vi "纳清探头一键校准.vi"(4 "校准量程":u16, 5 "校准方式":u16, 6 "MB_Master输入":refnum<class "MB_Master.lvclass">, 7 "探头":T1(ring), 8 "error in (no error)":errorcluster caption="错误输入（无错误）", 9 "标液三":cluster{"标准值":sgl, "检测值":sgl, "原始值":sgl}, 10 "标液二":cluster{"标准值":sgl, "检测值":sgl, "原始值":sgl}, 11 "标液一":cluster{"标准值":sgl, "检测值":sgl, "原始值":sgl}) -> (0 "error out":errorcluster caption="错误输出")   [LabVIEW 2016, in "斯坦道多参数.lvlib"]
uses:
  <vilib>/Plasmionique/MB Master/MB_Master/MB_Master.lvclass
  <vilib>/Plasmionique/MB Master/MB Master.lvlib
panel:
  out "数组":u16[](array[numeric]) format="%04x"
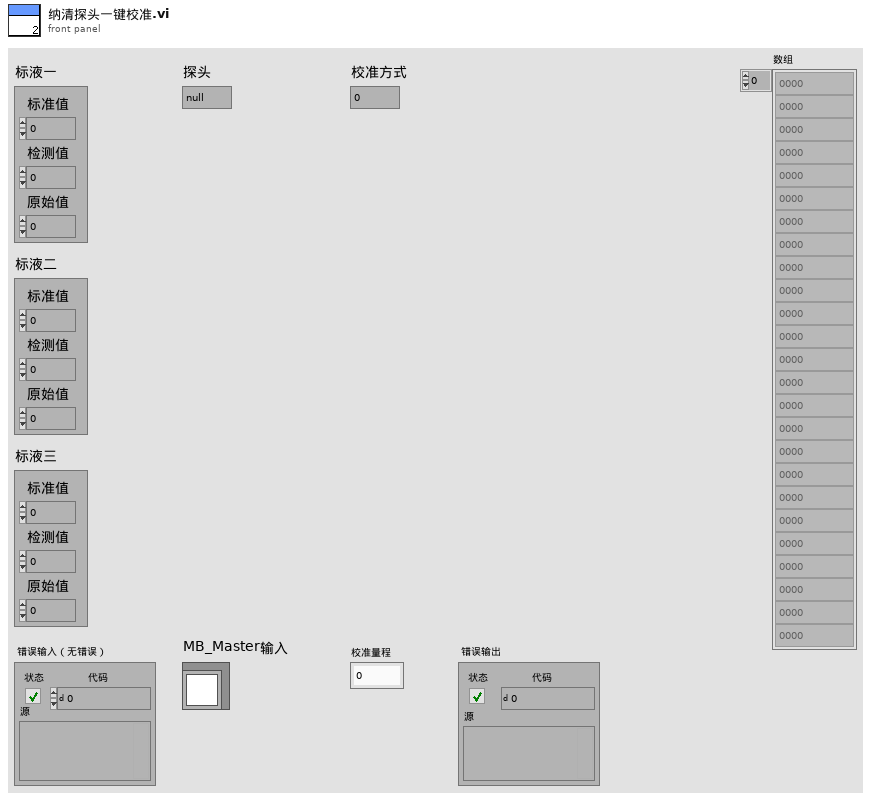
[diagram p1: front panel]
types:
  T1 = enum16{"null", "pH", "DO", "浊度", "电导率", "叶绿素a", "藻密度", "氨氮"}
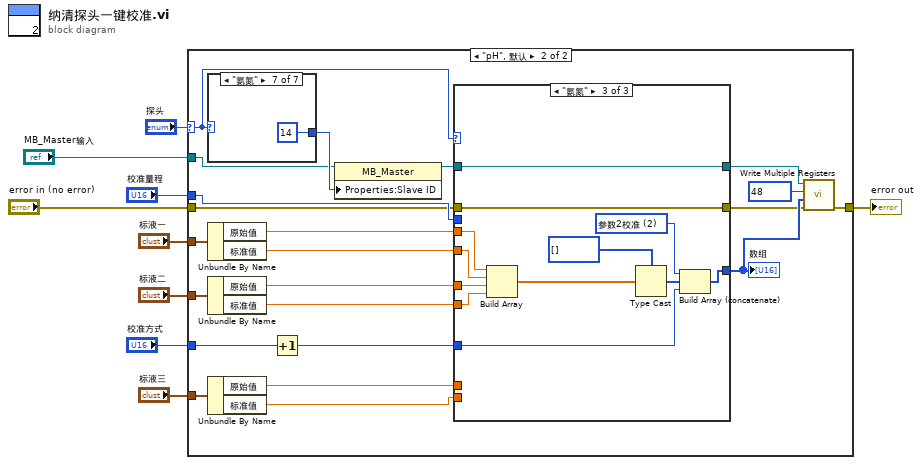
[diagram p0: block diagram]
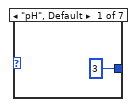
[diagram p3: hidden frame]
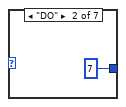
[diagram p4: hidden frame]
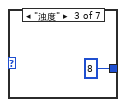
[diagram p5: hidden frame]
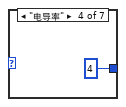
[diagram p6: hidden frame]
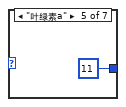
[diagram p7: hidden frame]
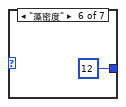
[diagram p8: hidden frame]
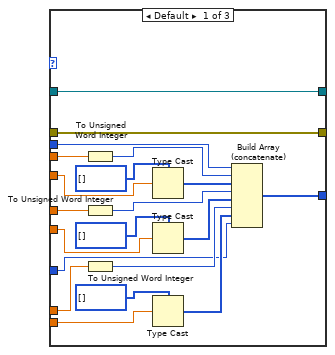
[diagram p9: hidden frame]
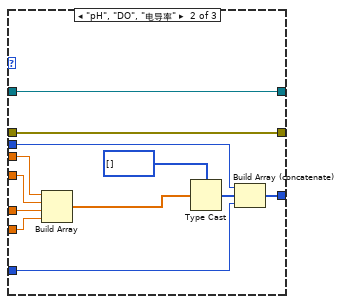
[diagram p10: hidden frame]
diagram:
  n1 = case shown="\"pH\", 默认" "探头" {
    selector: "探头" -> [_ w17]
    tunnel: "error in (no error)" -> [w10 w12]
    tunnel: [w10 w32] -> w8
    tunnel: "标液一" -> [_ w31]
    tunnel: "标液二" -> [_ w30]
    tunnel: "标液三" -> [_ w29]
    tunnel: "校准量程" -> [_ w22]
    tunnel: "校准方式" -> [_ w21]
    tunnel: "MB_Master输入" -> [_ w15]
    frame "null" {
    }
    frame "pH", Default {
      n2 = case shown="\"氨氮\"" w17 {
        tunnel: [3 7 8 4 11 12 14] -> w19
        frame "pH", Default {
        }
        frame "DO" {
        }
        frame "浊度" {
        }
        frame "电导率" {
        }
        frame "叶绿素a" {
        }
        frame "藻密度" {
        }
        frame "氨氮" {
        }
      }
      n3 = Unbundle By Name(w31) -> ("原始值"=w28:sgl, "标准值"=w25:sgl)
      n4 = Unbundle By Name(w30) -> ("原始值"=w27:sgl, "标准值"=w24:sgl)
      n5 = Unbundle By Name(w29) -> ("原始值"=w26:sgl, "标准值"=w23:sgl)
      n6 = Increment(x=w21) -> (x+1=w20:u16)
      n7 = property class="MB_Master"(reference=w15, "Properties:Slave ID"=w19) -> (reference out=w14:refnum<class "MB_Master.lvclass">)  [unwired: 1 in, 1 out]
      n8 = case shown="\"氨氮\"" w17 {
        tunnel: w28 -> [w59 w70 w82]
        tunnel: [w55 w64 w76] -> w16
        tunnel: w27 -> [w54 w68 w80]
        tunnel: w26 -> [w48 _ _]
        tunnel: w25 -> [w56 w69 w81]
        tunnel: w24 -> [w52 w67 w79]
        tunnel: w23 -> [w45 _ _]
        tunnel: w22 -> [w43 w63 _]
        tunnel: w20 -> [w42 w62 w75]
        tunnel: w14 -> [w41 w61 w73]
        tunnel: [w41 w61 w73] -> w13
        tunnel: w12 -> [w40 w60 w74]
        tunnel: [w40 w60 w74] -> w11
        frame Default {
          n9 = To Unsigned Word Integer(number=w59) -> (unsigned 16bit integer=w58:u16)
          n10 = To Unsigned Word Integer(number=w54) -> (unsigned 16bit integer=w50:u16)
          n11 = To Unsigned Word Integer(number=w48) -> (unsigned 16bit integer=w47:u16)
          n12 = Type Cast(type=u16[] [], x=w56) -> (*(type *) &x=w51:u16[])
          n13 = Type Cast(type=u16[] [], x=w52) -> (*(type *) &x=w49:u16[])
          n14 = Type Cast(type=u16[] [], x=w45) -> (*(type *) &x=w44:u16[])
          n15 = Build Array (concatenate)(w43, w58, w51, w50, w49, w47, w44, w42) -> (w55:u16[])
        }
        frame "pH", "DO", "电导率" {
          n16 = Build Array(w70, w69, w68, w67) -> (w66:sgl[])
          n17 = Type Cast(type=u16[] [], x=w66) -> (*(type *) &x=w65:u16[])
          n18 = Build Array (concatenate)(w63, w65, w62) -> (w64:u16[])
        }
        frame "氨氮" {
          w72 = u16 2 items=["参数1校准"=1, "参数2校准"=2, "参数3校准"=3, "参数4校准"=4] ("校准参数类型")
          n19 = Build Array(w82, w81, w80, w79) -> (w78:sgl[])
          n20 = Type Cast(type=u16[] [], x=w78) -> (*(type *) &x=w77:u16[])
          n21 = Build Array (concatenate)(w72, w77, w75) -> (w76:u16[])
        }
      }
      "数组" <- w16
      n22 = call <vilib>:"Write Multiple Registers.vi"("error in (no error)"=w11, "values"=w16, "starting address"=u16 48, "MB session in"=w13) -> ("error out"=w32:errorcluster)  [unwired: 6 in, 1 out]
    }
  }
  "error out" <- w8
